vi "Create.vi"(8 "error in (no error)":errorcluster) -> (0 "error out":errorcluster, 3 "Mock Class Generator out":refnum<class "Mock Error Handler Interface.lvclass">)   [LabVIEW 2020, in "Mock Error Handler Interface.lvclass"]
doc: "Create an instance of the mock class."
uses:
  Mock Error Handler Interface.lvclass
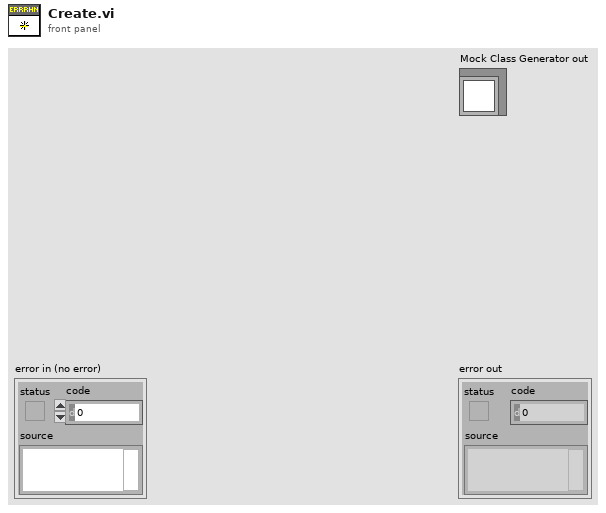
[diagram p1: front panel]
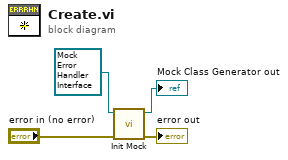
[diagram p0: block diagram]
diagram:
  n1 = call-dynamic "Init Mock.vi"("error in (no error)"="error in (no error)", "Mock In"=refnum<class "Mock Error Handler Interface.lvclass"> refnum ("Mock in")) -> ("error out"=→"error out":errorcluster, "Mock Out"=→"Mock Class Generator out":refnum<class "Mock Error Handler Interface.lvclass">)  [unwired: 8 in]
